vi "CALC_FUNC_STAT_STAT_ON_OFF.vi"(0 "VISA IN":refnum<visa-resource-name>, 1 "Display Trace Statistics ON/OFF":bool, 5 "error in":errorcluster, 7 "Channel":i32) -> (14 "VISA Out":refnum<visa-resource-name>, 19 "error out":errorcluster)   [LabVIEW 2018, in "PNA-X.lvlib"]
doc: "CALCulate<cnum>:FUNCtion:STATistics[:STATe] <ON|OFF> \n(Read-Write) Displays and hides the trace statistics (peak-to-peak, mean, standard deviation) on the \nscreen. \nThe analyzer will display either measurement statistics or Filter Bandwidth statistics; not both. \nSee Critical Note \nParameters \n<cnum> Channel number of the measurement. There must be a selected measurement \non that channel. If unspecified, <cnum> is set to 1. \n<ON|OFF> ON - Displays trace statistics \nOFF - Hides trace statistics \nExamples CALC:FUNC:STAT ON \ncalculate2:function:statistics:state off \nQuery Syntax CALCulate<cnum>:FUNCtion:STATistics[:STATe]? \nReturn Type Boolean (1 = ON, 0 = OFF) \nDefault OFF (0)"
uses:
  PNA-X.lvlib
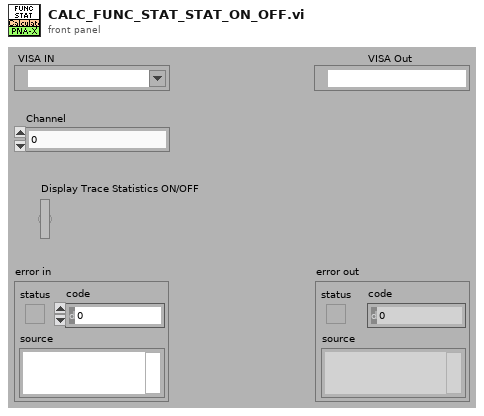
[diagram p1: front panel]
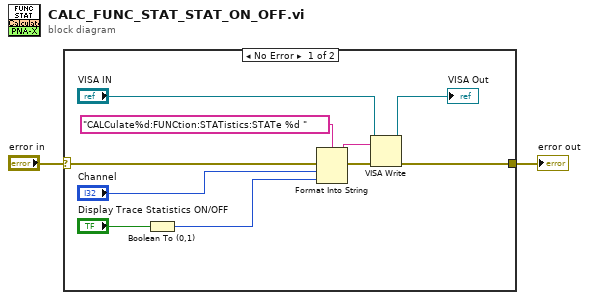
[diagram p0: block diagram]
diagram:
  n1 = case shown="No Error" "error in" {
    selector: "error in" -> [w12 w13]
    tunnel: [w7 w13] -> w1
    frame No Error {
      n2 = Boolean To (0,1)(Boolean="Display Trace Statistics ON/OFF") -> (0, 1=w3:i16)
      n3 = Format Into String(format string="CALCulate%d:FUNCtion:STATistics:STATe %d " ("Cmdline"), error in=w12, "Channel", w3) -> (resulting string=w10:string, error out=w11:errorcluster)  [unwired: 1 in]
      n4 = VISA Write(VISA resource name="VISA IN", write buffer=w10, error in (no error)=w11) -> (VISA resource name out=→"VISA Out":refnum<visa-resource-name>, error out=w7:errorcluster)  [unwired: 1 out]
    }
    frame Error {
    }
  }
  "error out" <- w1
